vi "RedisTabExecute.vi"(8 "Type":enum16{"Subscribe", "LPop", "Stream"}(ring), 9 "RedisTabQueue":refnum<queue>, 10 "RedisTabCondition":string="RedisKey@127.0.0.1:6379", 11 "RedisTabName":string="RedisKey") -> ()   [LabVIEW 2020]
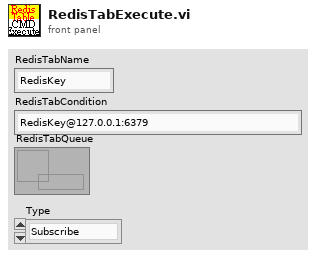
[diagram p1: front panel]
types:
  T1 = cluster{"Command":string, "Parameter":string, "queue out":refnum<queue>}
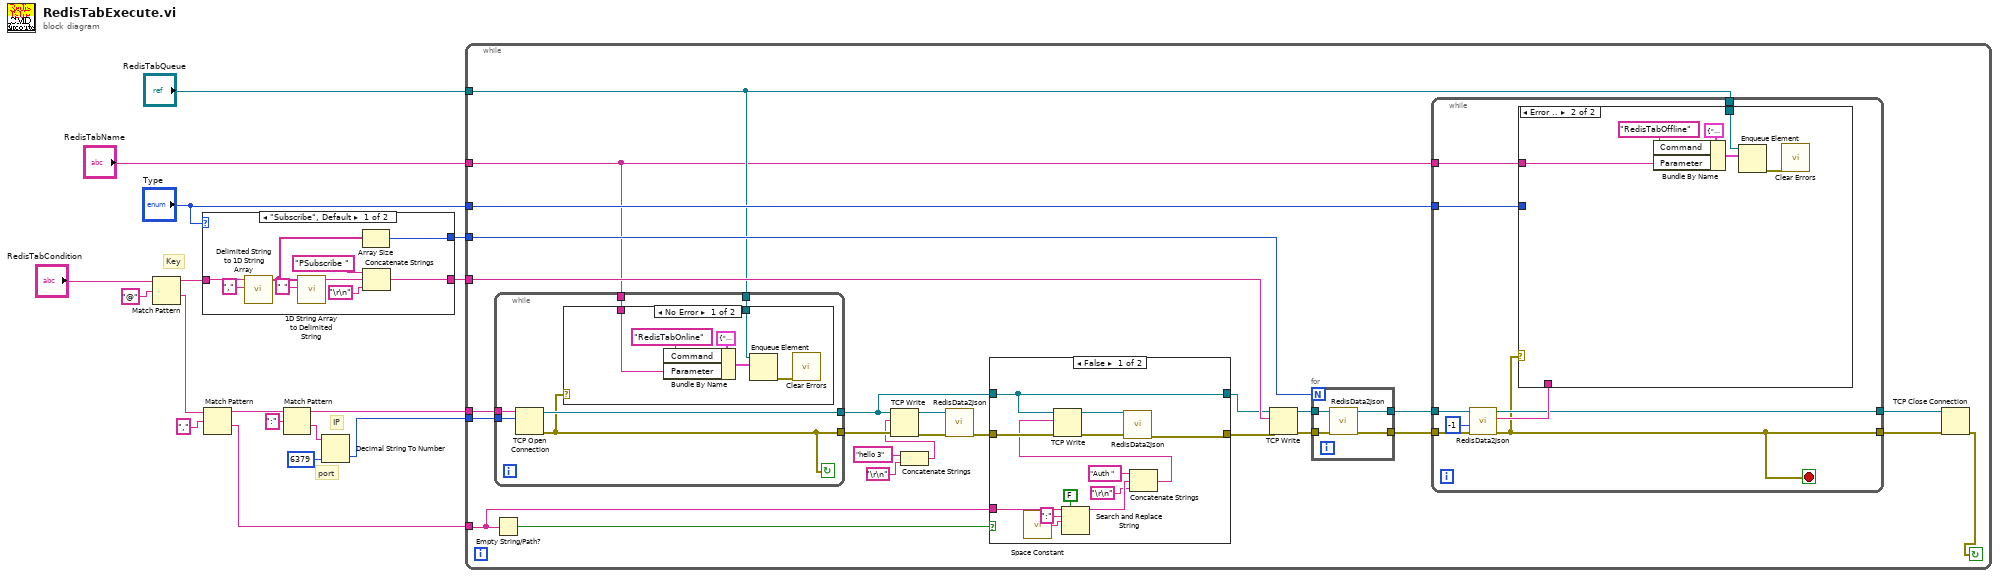
[diagram p0: block diagram]
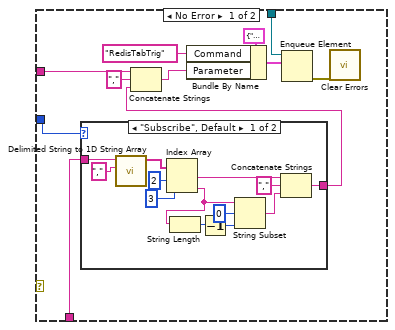
[diagram p3: hidden frame]
diagram:
  # "port"
  # "IP"
  # "Key"
  n1 = Match Pattern(string="RedisTabCondition", regular expression="@") -> (before substring=w15:string, after substring=w3:string)  [unwired: 1 in, 2 out]
  n2 = case shown="\"Subscribe\", Default" "Type" {
    tunnel: w15 -> [w25 _]
    tunnel: [w20 _] -> w9
    tunnel: [w18 _] -> w8
    frame "Subscribe", Default {
      n3 = call <vilib>:"Delimited String to 1D String Array.vi"("delimiter"=",", "delimited string"=w25) -> ("string array"=w19:string[])  [unwired: 9 in]
      n4 = call <vilib>:"1D String Array to Delimited String.vi"("delimiter"=" ", "string array"=w19) -> ("delimited string"=w22:string)  [unwired: 9 in]
      n5 = Array Size(array=w19) -> (size(s)=w18:i32)
      n6 = Concatenate Strings("PSubscribe " ("string"), w22, "\r\n") -> (w20:string)
    }
    frame "LPop" {
    }
  }
  n7 = Match Pattern(string=w3, regular expression=",") -> (before substring=w2:string, after substring=w1:string)  [unwired: 1 in, 2 out]
  n8 = Match Pattern(string=w2, regular expression=":") -> (before substring=w13:string, after substring=w12:string)  [unwired: 1 in, 2 out]
  n9 = Decimal String To Number(string=w12, default (0L)=u16 6379 ("remote port or service name")) -> (number=w10:u16)  [unwired: 1 in, 1 out]
  n10 = while {
    tunnel: w13 -> [w52]
    tunnel: w10 -> [w51]
    tunnel: w9 -> [w50]
    tunnel: w8 -> [w41]
    tunnel: "RedisTabQueue" -> [w34]
    tunnel: "RedisTabName" -> [w33]
    tunnel: "Type" -> [w38]
    tunnel: w1 -> [w27]
    stop <- w35 continue-if-true
    n11 = while {
      tunnel: w52 -> [w112]
      tunnel: w51 -> [w111]
      tunnel: [w109] -> w47
      tunnel: [w110] -> w32
      tunnel: w34 -> [w108]
      tunnel: w33 -> [w107]
      stop <- w109 continue-if-true
      n12 = TCP Open Connection(address=w112, remote port or service name=w111) -> (connection ID=w110:refnum<k5>, error out=w109:errorcluster)  [unwired: 3 in]
      n13 = case shown="No Error" w109 {
        tunnel: w108 -> [w113 _]
        tunnel: w107 -> [w115 _]
        frame No Error {
          n14 = Bundle By Name(cluster=T1 {"Command"="", "Parameter"="", "queue out"=refnum} ("element"), "Command"="RedisTabOnline", "Parameter"=w115) -> (w118:T1)
          n15 = Enqueue Element(queue=w113, element=w118) -> (error out=w116:errorcluster)  [unwired: 2 in, 2 out]
          n16 = call <vilib>:"Clear Errors.vi"("error in (no error)"=w116) -> ()  [unwired: 5 in, 2 out]
        }
        frame Error {
        }
      }
    }
    n17 = Empty String/Path?(string/path=w27) -> (empty?=w28:bool)
    n18 = Concatenate Strings("hello 3" ("string"), "\r\n") -> (w44:string)
    n19 = TCP Write(connection ID=w32, data in=w44, error in (no error)=w47) -> (connection ID out=w42:refnum<k5>, error out=w43:errorcluster)  [unwired: 1 in, 1 out]
    n20 = call "RedisData2Json.vi"("error in"=w43, "RedisSession"=w42) -> ("error out"=w30:errorcluster)  [unwired: 6 in, 3 out]
    n21 = case shown="False" w28 {
      tunnel: w32 -> [w59 w67]
      tunnel: [w59 w67] -> w31
      tunnel: w30 -> [w65 w66]
      tunnel: [w57 w66] -> w29
      tunnel: w27 -> [w61 _]
      frame False {
        n22 = call <vilib>:"Space Constant.vi"() -> ("String"=w63:string)
        n23 = Search and Replace String(replace all?=FALSE ("replace all? (F)"), input string=w61, search string=":", replace string=w63) -> (result string=w55:string)  [unwired: 4 in, 3 out]
        n24 = Concatenate Strings("Auth " ("string"), w55, "\r\n") -> (w53:string)
        n25 = TCP Write(connection ID=w59, data in=w53, error in (no error)=w65) -> (connection ID out=w60:refnum<k5>, error out=w58:errorcluster)  [unwired: 1 in, 1 out]
        n26 = call "RedisData2Json.vi"("error in"=w58, "RedisSession"=w60) -> ("error out"=w57:errorcluster)  [unwired: 6 in, 3 out]
      }
      frame True {
      }
    }
    n27 = TCP Write(connection ID=w31, data in=w50, error in (no error)=w29) -> (connection ID out=w49:refnum<k5>, error out=w48:errorcluster)  [unwired: 1 in, 1 out]
    n28 = for {
      N: w41 -> [_]
      tunnel: w49 -> [w122]
      tunnel: [w119] -> w40
      tunnel: w48 -> [w121]
      tunnel: [w120] -> w39
      n29 = call "RedisData2Json.vi"("error in"=w121, "RedisSession"=w122) -> ("error out"=w120:errorcluster, "RedisSession"=w119:refnum<k5>)  [unwired: 6 in, 2 out]
    }
    n30 = while {
      tunnel: w34 -> [w73]
      tunnel: w33 -> [w72]
      tunnel: w38 -> [w71]
      tunnel: w40 -> [w76]
      tunnel: [w69] -> w37
      tunnel: w39 -> [w75]
      tunnel: [w68] -> w36
      stop <- w68 stop-if-true
      n31 = call "RedisData2Json.vi"("error in"=w75, "TimeOut"=-1, "RedisSession"=w76) -> ("error out"=w68:errorcluster, "JSON"=w70:string, "RedisSession"=w69:refnum<k5>)  [unwired: 5 in, 1 out]
      n32 = case shown="Error .." w68 {
        tunnel: w73 -> [w87 w106]
        tunnel: w72 -> [w82 w101]
        tunnel: w71 -> [w80 _]
        tunnel: w70 -> [w79 _]
        frame No Error {
          n33 = case shown="\"Subscribe\", Default" w80 {
            tunnel: w79 -> [w100 _]
            tunnel: [w93 _] -> w78
            frame "Subscribe", Default {
              n34 = call <vilib>:"Delimited String to 1D String Array.vi"("delimiter"=",", "delimited string"=w100) -> ("string array"=w98:string[])  [unwired: 9 in]
              n35 = Index Array(array=w98, index #1=2 ("index"), index #2=3 ("index")) -> (element #1=w95:string, element #2=w91:string)
              n36 = String Length(string=w91) -> (length=w90:i32)
              n37 = Decrement(x=w90) -> (x-1=w89:i32)
              n38 = String Subset(string=w91, offset (0)=0, length (rest)=w89) -> (substring=w88:string)
              n39 = Concatenate Strings(w95, "," ("string"), w88) -> (w93:string)
            }
            frame "LPop" {
            }
          }
          n40 = Concatenate Strings(w82, "," ("string"), w78) -> (w83:string)
          n41 = Bundle By Name(cluster=T1 {"Command"="", "Parameter"="", "queue out"=refnum} ("element"), "Command"="RedisTabTrig", "Parameter"=w83) -> (w85:T1)
          n42 = Enqueue Element(queue=w87, element=w85) -> (error out=w77:errorcluster)  [unwired: 2 in, 2 out]
          n43 = call <vilib>:"Clear Errors.vi"("error in (no error)"=w77) -> ()  [unwired: 5 in, 2 out]
        }
        frame Error {
          n44 = Bundle By Name(cluster=T1 {"Command"="", "Parameter"="", "queue out"=refnum} ("element"), "Command"="RedisTabOffline", "Parameter"=w101) -> (w104:T1)
          n45 = Enqueue Element(queue=w106, element=w104) -> (error out=w102:errorcluster)  [unwired: 2 in, 2 out]
          n46 = call <vilib>:"Clear Errors.vi"("error in (no error)"=w102) -> ()  [unwired: 5 in, 2 out]
        }
      }
    }
    n47 = TCP Close Connection(connection ID=w37, error in (no error)=w36) -> (error out=w35:errorcluster)  [unwired: 1 in, 1 out]
  }
